vi "PH_SSAC.Calc BG-Mean.vi"(0 "i ref in":refnum<vi>, 5 "error out":errorcluster) -> (14 "i ref out":refnum<vi>, 17 "BG Mean Value [Pixel]":dbl, 19 "error out":errorcluster)   [LabVIEW 2014, in "PH_SSAC.lvlib"]
doc: "This VI calculates the mean value inside the background frame."
uses:
  PH_SSAC.lvlib
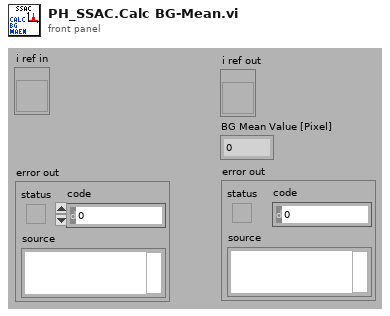
[diagram p1: front panel]
types:
  T1 = typedef "PH_SSAC.lvlib/PH_SSAC.i attribute.ctl" = cluster{"GUI Refs":cluster{"Delete":refnum<vi>, "Global On":refnum<vi>, "Cam Source":refnum<vi>, "Frame Main Signal":refnum<vi>, "Frame Background":refnum<vi>, "dt (Gauss smooth)":refnum<vi>, "Calibration Factor":refnum<vi>, "Background acquire":refnum<vi>, "Threshold":refnum<vi>, "Time evolution of mean pulse duration":refnum<vi>, "Mean Pulse Duration":refnum<vi>, "Main signal":refnum<vi>, "Current Pulse Duration":refnum<vi>, "Processed":refnum<vi>, "Saturation":refnum<vi>, "# for Average":refnum<vi>, "Position":refnum<vi>, "BG Status":refnum<vi>, "Save BG data":refnum<vi>, "Read BG Data":refnum<vi>, "Background Calibration Data":refnum<vi>}, "Images":cluster{"OP Image":T2, "GUI Image":T2, "PSDB Image":T2}, "Global On?":bool, "Frame Main":cluster{"x":u32, "dx":u32, "y":u32, "dy":u32}, "Frame Background":cluster{"x":u32, "dx":u32, "y":u32, "dy":u32}, "dt [fs]":dbl, "Calibration Factor [fs/pixel]":dbl, "Threshold":dbl, "Time evolution of mean pulse duration [fs]":dbl[], "Main Signal":cluster{"Time for Main":dbl[], "Signal":dbl[]}, "Processed":bool, "Current Pulse Duration [fs]":dbl, "# for Average":i32, "Position":i32, "Pulse Durations [fs]":dbl[], "BG":cluster{"Acquire?":bool, "Background Calibration Data":T3, "Save Data":bool}}
  T2 = typedef "IMAQ Image.ctl" = refnum<image>
  T3 = typedef "PH_SSAC.lvlib/PH_SSAC.Background Data.ctl" = cluster{"Date":string, "Time":string, "Frame Main":cluster{"x":u32, "dx":u32, "y":u32, "dy":u32}, "dt [fs]":dbl, "Calibration Factor [fs/pixel]":dbl, "Signal":dbl[], "Frame Background":cluster{"x":u32, "dx":u32, "y":u32, "dy":u32}}
  T4 = cluster{"Left":i32, "Top":i32, "Right":i32, "Bottom":i32}
  T5 = typedef "Image Type" = u32
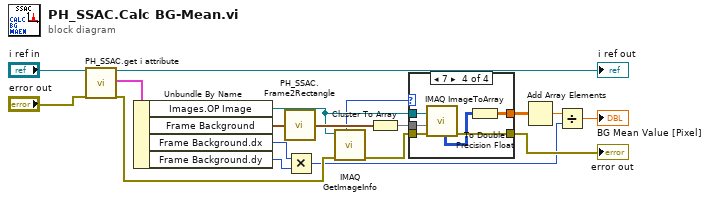
[diagram p0: block diagram]
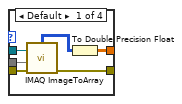
[diagram p2: hidden frame]
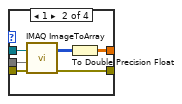
[diagram p3: hidden frame]
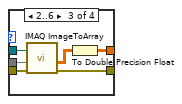
[diagram p4: hidden frame]
diagram:
  n1 = call "PH_SSAC.get i attribute.vi"("i ref in"="i ref in", "error in (no error)"="error out") -> ("i ref out"=→"i ref out":refnum<vi>, "i attribute"=w14:T1, "error out"=w18:errorcluster)  [unwired: 15 in]
  n2 = Unbundle By Name(w14) -> ("Images.OP Image"=w2:T2, "Frame Background"=w6:cluster{"x":u32, "dx":u32, "y":u32, "dy":u32}, "Frame Background.dx"=w10:u32, "Frame Background.dy"=w11:u32)
  n3 = call "PH_SSAC.Frame2Rectangle.vi"("Frame"=w6) -> ("Rectangle"=w5:T4)
  n4 = Multiply(x=w10, y=w11) -> (x*y=w9:u32)
  n5 = call "IMAQ GetImageInfo"("error in (no error)"=w18, "Image"=w2) -> ("error out"=w3:errorcluster, "Image Type"=w1:T5)  [unwired: 2 in, 6 out]
  n6 = Cluster To Array(cluster=w5) -> (array=w4:i32[])
  n7 = case shown="7" w1 {
    tunnel: [w24 w30 w36 w42] -> w7
    tunnel: [w23 w29 w35 w41] -> w12
    tunnel: w4 -> [w22 w28 w34 w40]
    tunnel: w3 -> [w21 w27 w33 w39]
    tunnel: w2 -> [w20 w26 w32 w38]
    frame Default {
      n8 = call "IMAQ ImageToArray"("error in (no error)"=w21, "Optional Rectangle"=w22, "Image"=w20) -> ("error out"=w23:errorcluster, "Image Pixels (U8)"=w19:u8[][])  [unwired: 1 in, 3 out]
      n9 = To Double Precision Float(number=w19) -> (double precision float=w24:dbl[][])
    }
    frame 1 {
      n10 = call "IMAQ ImageToArray"("error in (no error)"=w27, "Optional Rectangle"=w28, "Image"=w26) -> ("error out"=w29:errorcluster, "Image Pixels (I16)"=w25:i16[][])  [unwired: 1 in, 3 out]
      n11 = To Double Precision Float(number=w25) -> (double precision float=w30:dbl[][])
    }
    frame 2..6 {
      n12 = call "IMAQ ImageToArray"("error in (no error)"=w33, "Optional Rectangle"=w34, "Image"=w32) -> ("Image Pixels (Float)"=w31:sgl[][], "error out"=w35:errorcluster)  [unwired: 1 in, 3 out]
      n13 = To Double Precision Float(number=w31) -> (double precision float=w36:dbl[][])
    }
    frame 7 {
      n14 = call "IMAQ ImageToArray"("error in (no error)"=w39, "Optional Rectangle"=w40, "Image"=w38) -> ("Image Pixels (U16)"=w37:u16[][], "error out"=w41:errorcluster)  [unwired: 1 in, 3 out]
      n15 = To Double Precision Float(number=w37) -> (double precision float=w42:dbl[][])
    }
  }
  "error out" <- w12
  n16 = Add Array Elements(numeric array=w7) -> (sum=w8:dbl)
  n17 = Divide(x=w8, y=w9) -> (x/y=→"BG Mean Value [Pixel]":dbl)
